vi "Inverse Real FFT.vi"(10 "shift?":bool, 11 "FFT {X}":cdb[](array[numeric])) -> (0 "error":i32, 3 "X":dbl[](array[numeric]))   [LabVIEW 2010, in "NI_AALPro.lvlib"]
doc: "Computes the inverse discrete Fourier transform (IDFT) of the input sequence <B>FFT {X}</B>. You must manually select the polymorphic instance you want to use."
uses:
  NI_AALPro.lvlib
  lvanlys.dll
panel:
  # "Inverse Real FFT"
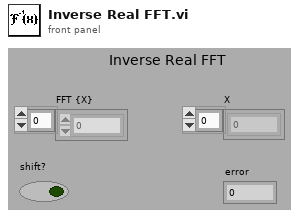
[diagram p1: front panel]
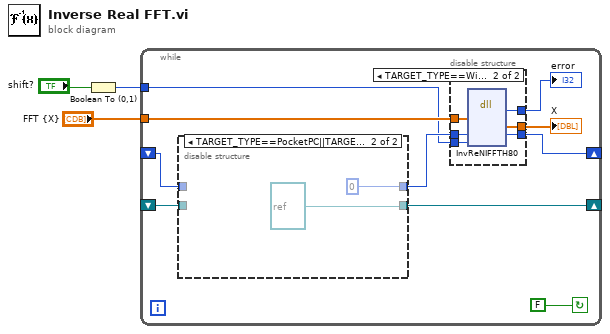
[diagram p0: block diagram]
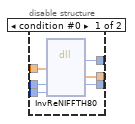
[diagram p2: hidden frame]
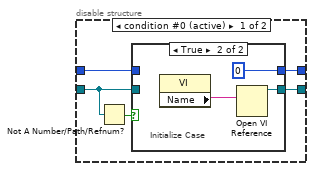
[diagram p3: hidden frame]
diagram:
  n1 = Boolean To (0,1)(Boolean="shift?") -> (0, 1=w1:i16)
  n2 = while {
    shift-left: _ -> [w7]
    shift-right: [w9] -> _
    tunnel: "FFT {X}" -> [w13]
    shift-right: [w5] -> _
    shift-left: _ -> [w6]
    tunnel: w1 -> [w4]
    stop <- FALSE continue-if-true
    n3 = disable-structure shown="TARGET_TYPE==PocketPC||TARGET_TYPE==PalmOS||TARGET_TYPE==FPGA||TARGET_TYPE==Embedded" {
      disable-tunnel: w6 -> [w28 _]
      disable-tunnel: [w29 refnum<vi> refnum ("VI Refnum")] -> w5
      disable-tunnel: w7 -> [w27 _]
      disable-tunnel: [w26 0 ("t")] -> w8
      frame condition #0 (active) {
        n4 = Not A Number/Path/Refnum?(number/path/refnum=w28) -> (NaN/Path/Refnum?=w30:bool)
        n5 = case shown="True" w30 {
          tunnel: [w32 w34] -> w29
          tunnel: w28 -> [w32 _]
          tunnel: w27 -> [w31 _]
          tunnel: [w31 0 ("error")] -> w26
          frame False {
          }
          frame True {
            # "Initialize Case"
            n6 = property class="VI"() -> ("Name"=w33:string)  [unwired: 2 in, 2 out]
            n7 = Open VI Reference(vi path=w33) -> (vi reference=w34:refnum<vi>)  [unwired: 5 in, 1 out]
          }
        }
      }
      frame condition #1 {
      }
    }
    n8 = disable-structure shown="TARGET_TYPE==Windows||TARGET_TYPE==Mac||TARGET_TYPE==Unix" {
      disable-tunnel: w13 -> [w19 w25]
      disable-tunnel: [w18 w24] -> w12
      disable-tunnel: [w17 w23] -> w11
      disable-tunnel: [w16 w22] -> w9
      disable-tunnel: w8 -> [w15 w21]
      disable-tunnel: w4 -> [w14 w20]
      frame condition #0 {
        n9 = dll-call lib="C:/Program Files/National Instruments/LabVIEW 2010/resource/lvanlys.dll" fn="InvReNIFFTH80"("xH"=w19, "tbl"=w15, "shift"=w14) -> ("return type"=w18:i32, "yH"=w17:dbl[], "tbl"=w16:i32)  [unwired: 6 in, 2 out]
      }
      frame condition #1 (active) {
        n10 = dll-call lib="C:/Program Files/National Instruments/LabVIEW 2010/resource/lvanlys.dll" fn="InvReNIFFTH80"("xH"=w25, "tbl"=w21, "shift"=w20) -> ("return type"=w24:i32, "yH"=w23:dbl[], "tbl"=w22:i64)  [unwired: 6 in, 2 out]
      }
    }
    "X" <- w11
    "error" <- w12
  }
